vi "test_ccd_gain.vi"(8 "error in":errorcluster, 11 "CCD in":refnum<class "CCD.lvclass">) -> (0 "error out":errorcluster, 3 "CCD out":refnum<class "CCD.lvclass">)   [LabVIEW 2023, in "horiba.test.lvlib"]
uses:
  horiba.test.lvlib
  Classes/CCD/CCD.lvclass
  C:/Projects/Horiba/horiba-labview-sdk/Source/Classes/GenericDevice/GenericDevice.lvclass
  <vilib>/addons/_JKI Toolkits/Caraya/classes/Assert/Assert Equal Value and Type_Variant.vi
  <vilib>/addons/_JKI Toolkits/Caraya/classes/Test/Test.lvclass
  <vilib>/addons/_JKI Toolkits/Caraya/classes/Assert/Assert.lvclass
  <userlib>/_OpenG.lib/lvdata/lvdata.llb/openg_variant.lvlib
panel:
  # "Connector Pane"
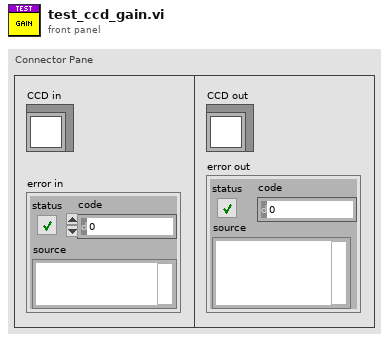
[diagram p1: front panel]
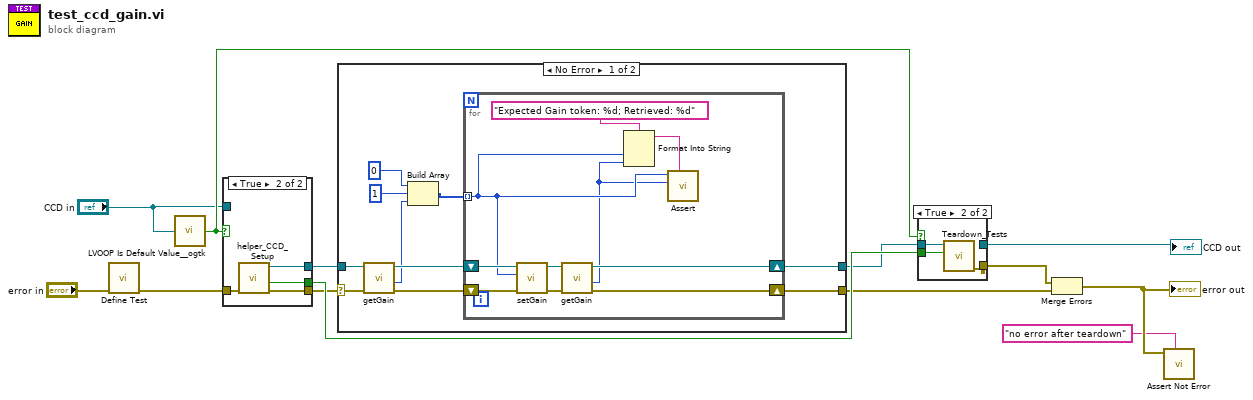
[diagram p0: block diagram]
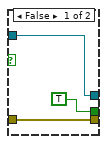
[diagram p3: hidden frame]
diagram:
  n1 = call <vilib>:"Define Test.vi"("error in (no error)"="error in") -> ("error out"=w8:errorcluster)  [unwired: 9 in, 1 out]
  n2 = call <userlib>:"LVOOP Is Default Value__ogtk.vi"("Object"="CCD in") -> ("Is Default Value?"=w9:bool)
  n3 = case shown="True" w9 {
    tunnel: w8 -> [w15 w20]
    tunnel: [w15 w19] -> w4
    tunnel: [w16 w18] -> w6
    tunnel: [TRUE ("Module Was Already Running?") w17] -> w10
    tunnel: "CCD in" -> [w16 _]
    frame False {
    }
    frame True {
      n4 = call "helper_CCD_Setup.vi"("error in"=w20) -> ("error out"=w19:errorcluster, "Module Was Already Running?"=w17:bool, "CCD out"=w18:refnum<class "CCD.lvclass">)  [unwired: 7 in, 1 out]
    }
  }
  n5 = case shown="No Error" w4 {
    selector: w4 -> [w30 w41]
    tunnel: [w27 w42] -> w5
    tunnel: w6 -> [w29 w42]
    tunnel: [w25 w41] -> w3
    frame No Error {
      n6 = call "getGain.vi"("error in (no error)"=w30, "CCD in"=w29) -> ("error out"=w26:errorcluster, "token"=w22:i32, "CCD out"=w28:refnum<class "CCD.lvclass">)  [unwired: 6 in, 1 out]
      n7 = Build Array(0 ("token"), 1 ("element"), w22) -> (w21:i32[])
      n8 = for {
        shift-right: [w37] -> w27
        shift-left: w28 -> [w38]
        shift-right: [w35] -> w25
        shift-left: w26 -> [w36]
        tunnel: w21 -> [w32] mode=indexing
        n9 = call "setGain.vi"("error in (no error)"=w36, "token"=w32, "CCD in"=w38) -> ("error out"=w40:errorcluster, "CCD out"=w39:refnum<class "CCD.lvclass">)  [unwired: 5 in, 2 out]
        n10 = call "getGain.vi"("error in (no error)"=w40, "CCD in"=w39) -> ("error out"=w35:errorcluster, "token"=w31:i32, "CCD out"=w37:refnum<class "CCD.lvclass">)  [unwired: 6 in, 1 out]
        n11 = Format Into String(format string="Expected Gain token: %d; Retrieved: %d", w32, w31) -> (resulting string=w34:string)  [unwired: 2 in, 1 out]
        n12 = call-poly <vilib>:"Assert.vi"("Label"=w34, "Y"=w31, "X"=w32) -> ()  [unwired: 7 in, 2 out]
      }
    }
    frame Error {
    }
  }
  n13 = case shown="True" w9 {
    tunnel: w5 -> [w43 w46]
    tunnel: [_ w45] -> w7
    tunnel: w10 -> [_ w44]
    tunnel: [w43 _] -> w1
    frame False {
    }
    frame True {
      n14 = call "Teardown_Tests.vi"("Module Was Already Running?"=w44, "horiba.lvlib:GenericDevice"=w46) -> ("error out"=w45:errorcluster)  [unwired: 8 in, 1 out]
    }
  }
  "CCD out" <- w1
  n15 = Merge Errors(w7, w3) -> (w12:errorcluster)
  "error out" <- w12
  n16 = call <vilib>:"Assert Not Error.vi"("Label"="no error after teardown", "Not Error?"=w12) -> ()  [unwired: 8 in, 2 out]
